vi "get-node-ids.vi"(11 "Graph in":refnum<class "Graph.lvclass">) -> (2 "node-ids":refnum<class "ID.lvclass">[](array[class]))   [LabVIEW 2020, in "graph.lvlib" / "Graph.lvclass"]
uses:
  Graph.lvclass
  ID/ID.lvclass
  Graph.lvclass/Graph.ctl
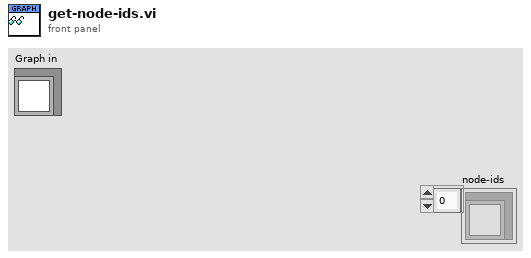
[diagram p1: front panel]
types:
  T1 = map{refnum<class "ID.lvclass">, refnum<class "Node.lvclass">}
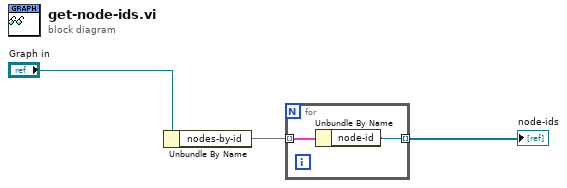
[diagram p0: block diagram]
diagram:
  n1 = Unbundle By Name("Graph in") -> ("nodes-by-id"=w1:T1)
  n2 = for {
    tunnel: w1 -> [w5] mode=indexing
    tunnel: [w4] -> w2 mode=indexing
    n3 = Unbundle By Name(w5) -> ("node-id"=w4:refnum<class "ID.lvclass">)
  }
  "node-ids" <- w2
